vi "Write AST.vi"(5 "AST":refnum<class "VI_AST.lvclass">, 9 "Diagram in":refnum<class "Diagram.lvclass">) -> (3 "Diagram out":refnum<class "Diagram.lvclass">)   [LabVIEW 2014, in "Diagram.lvclass"]
uses:
  Diagram.lvclass
  VI_AST/VI_AST.lvclass
  Diagram.lvclass/Diagram.ctl
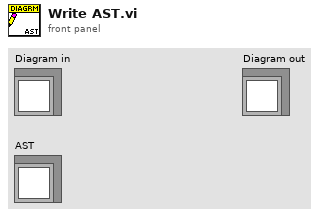
[diagram p1: front panel]
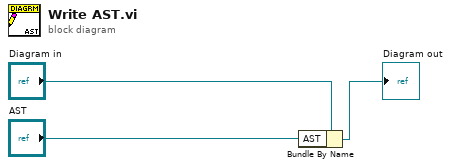
[diagram p0: block diagram]
diagram:
  n1 = Bundle By Name(cluster="Diagram in", "AST"="AST") -> (→"Diagram out":refnum<class "Diagram.lvclass">)
